vi "Hopper Loop.vi"   [LabVIEW 2016]
uses:
  Robot Global Data.vi
  <vilib>/Rock Robotics/WPI/Solenoid/Deprecated/WPI_SolenoidSetBool.vi
types:
  T1 = typedef "Intake Control Cluster.ctl" = cluster{"Intake Mode":T2, "Intake Auto Command":T3, "Intake Current Trip State":T4, "Gear slot open?":bool, "Engage traction for gear load?":bool, "Wings open?":bool}
  T2 = typedef "Intake Modes.ctl" = enum16{"Manual", "Auto"}
  T3 = typedef "Intake Auto States.ctl" = enum16{"Outake Ball", "Idle", "Load Ball"}
  T4 = typedef "Intake Trip States.ctl" = enum16{"Normal", "Backward Tripped", "Forward Tripped"}
  T5 = typedef "WPI_SolenoidDevRef.ctl" = cluster{"DevStatus":errorcluster, "Pneumatics Control Module":u8, "Forward Solenoid Channel":T6, "Reverse Solenoid Channel":T6}
  T6 = typedef "WPI_SolenoidChannel.ctl" = enum8{"Solenoid 0", "Solenoid 1", "Solenoid 2", "Solenoid 3", "Solenoid 4", "Solenoid 5", "Solenoid 6", "Solenoid 7", "Invalid"}
  T7 = typedef "Intake Status Cluster.ctl" = cluster{"Roller Power":dbl, "Intake Mode":T2, "Intake Auto State":T3, "Backward Tripped?":bool, "Forward Tripped?":bool, "Filling Hopper?":bool, "Intake Current Trip State":T4, "Getting Gear?":bool, "Gear Slot Open":bool, "Wings Open":bool}
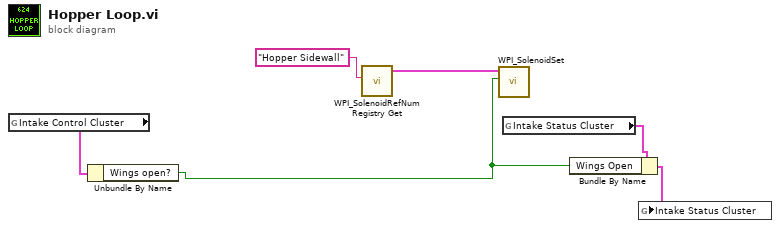
[diagram p0: block diagram]
diagram:
  n1 = global read "Robot Global Data.vi" "Intake Control Cluster"() -> (w2:T1)
  n2 = Unbundle By Name(w2) -> ("Wings open?"=w1:bool)
  n3 = call <vilib>:"WPI_SolenoidRefNum Registry Get.vi"("refnum name"="Hopper Sidewall") -> ("SolenoidDevRef"=w6:T5)  [unwired: 9 in, 1 out]
  n4 = call-poly <vilib>:"WPI_SolenoidSet.vi"("Value"=w1, "SolenoidDevRef"=w6) -> ()  [unwired: 8 in, 2 out]
  n5 = global read "Robot Global Data.vi" "Intake Status Cluster"() -> (w4:T7)
  n6 = Bundle By Name(cluster=w4, "Wings Open"=w1) -> (w3:T7)
  n7 = global write "Robot Global Data.vi" "Intake Status Cluster"(w3) -> ()
